vi "Create.vi"(8 "error in (no error)":errorcluster, 10 "Publish Q":refnum<queue>) -> (0 "error out":errorcluster, 3 "Telemetry API out":refnum<class "Telemetry API.lvclass">)   [LabVIEW 2020, in "VolatusTelemetry.lvlib" / "Telemetry API.lvclass"]
uses:
  Telemetry API.lvclass
  Telemetry API.lvclass/Telemetry API.ctl
  lv-protoc/LV-Proto/Message/Message.lvclass
  lv-vecto/Vecto/Group Data Type.ctl
  lv-vecto/VectoConfig/VectoConfig.lvlib
  Publish Group Data.ctl
  VolatusTelemetry.lvlib
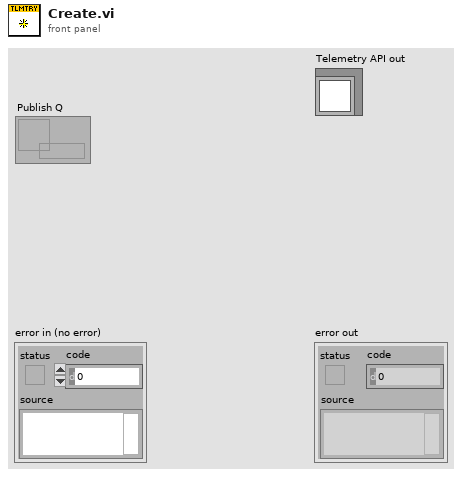
[diagram p1: front panel]
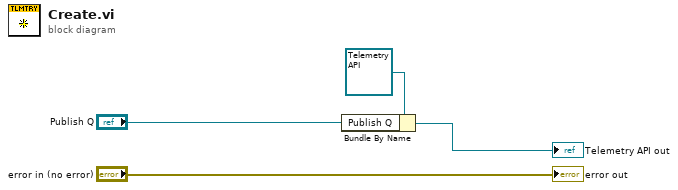
[diagram p0: block diagram]
diagram:
  n1 = Bundle By Name(cluster=refnum<class "Telemetry API.lvclass"> refnum ("Telemetry API in"), "Publish Q"="Publish Q") -> (→"Telemetry API out":refnum<class "Telemetry API.lvclass">)
  "error out" <- "error in (no error)"
